vi "DMR_OpenDevice.vi"(4 "device handle IN":i32) -> (0 "error code OUT":i32, 1 "device handle OUT":i32, 2 "driver handle OUT":i32)   [LabVIEW 2016]
doc: "Initialises a device.\n\nThis function will try to initialise the device associated with 'device handle IN'. On a successful call to this VI 'driver handle OUT' will contain a handle to the devices driver interface. This handle then can be used to call various driver functions or access and use device specific properties and objects.\n\nSee also:\nDMR_CloseDevice,\nDMR_GetDevice\n\nThe 'error code OUT' terminal will deliver 0 if successful or a negative error code otherwise. A list of valid error codes and their meaning can be found in the manual about this interface."
uses:
  mvDeviceManager.dll
panel:
  # "OUTPUT"
  # "INPUT"
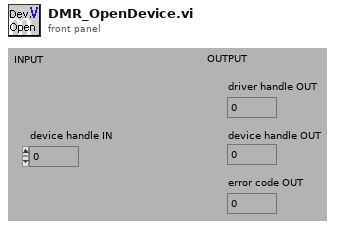
[diagram p1: front panel]
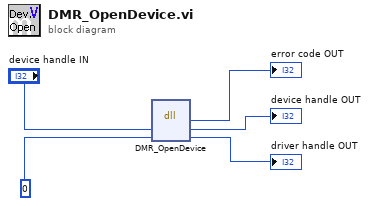
[diagram p0: block diagram]
diagram:
  n1 = dll-call lib="mvDeviceManager.dll" fn="DMR_OpenDevice"("hDev"="device handle IN", "phDrv"=0) -> (→"error code OUT":i32, "hDev"=→"device handle OUT":i32, "phDrv"=→"driver handle OUT":i32)  [unwired: 3 in, 2 out]
